vi "getResistance.vi"(5 "Uncertainty (%) Resistor":dbl=1.0, 6 "Uncertainty (%) Vin":dbl=1.0, 7 "Uncertainty (%) Vout":dbl=1.0, 8 "error in (no error)":errorcluster, 9 "V_in (V)":dbl=5.0, 10 "Resistor (ohms)":dbl=10000.0) -> (0 "error out":errorcluster, 2 "Uncertainty (%) Thermistor":dbl=3.0625, 3 "Resistance (ohms)":dbl=10000.0)   [LabVIEW 2013]
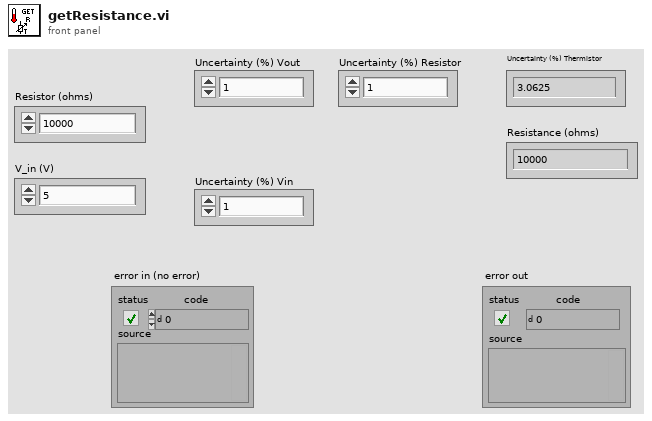
[diagram p1: front panel]
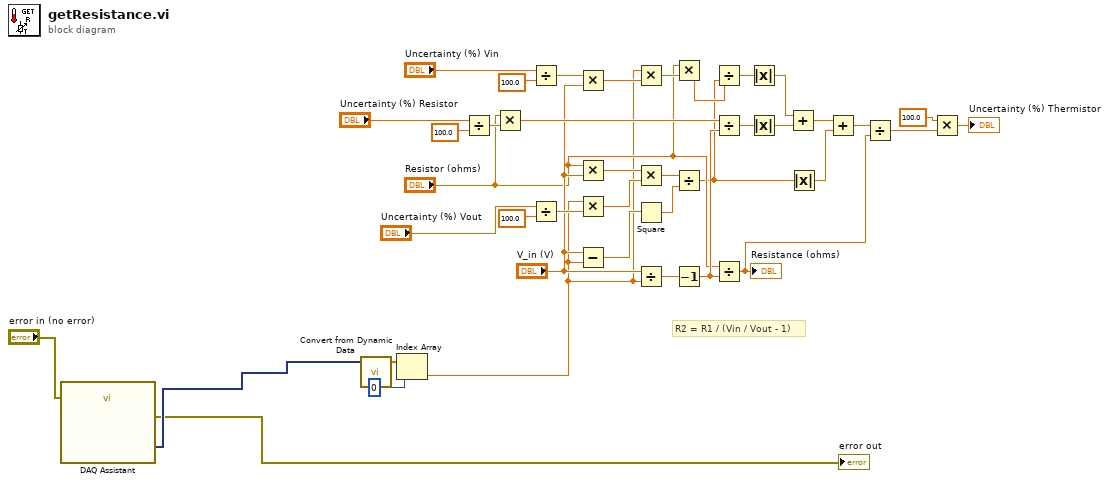
[diagram p0: block diagram]
diagram:
  # "R2 = R1 / (Vin / Vout - 1)"
  n1 = call "DAQ Assistant"("error in"="error in (no error)") -> ("data"=w2:dynamicdata, "error out"=→"error out":errorcluster)  [unwired: 16 in, 1 out]
  n2 = call "Convert from Dynamic Data"("Dynamic Data Type"=w2) -> ("Array"=w6:dbl[])  [unwired: 3 in]
  n3 = Index Array(array=w6, index=0) -> (element=w4:dbl)
  n4 = Divide(x="Uncertainty (%) Resistor", y=100.0) -> (x/y=w30:dbl)
  n5 = Multiply(x="Resistor (ohms)", y=w30) -> (x*y=w37:dbl)
  n6 = Divide(x="Uncertainty (%) Vin", y=100.0) -> (x/y=w22:dbl)
  n7 = Divide(x="Uncertainty (%) Vout", y=100.0) -> (x/y=w26:dbl)
  n8 = Multiply(x=w22, y="V_in (V)") -> (x*y=w21:dbl)
  n9 = Multiply(x="Resistor (ohms)", y="V_in (V)") -> (x*y=w35:dbl)
  n10 = Multiply(x=w4, y=w26) -> (x*y=w34:dbl)
  n11 = Subtract(x="V_in (V)", y=w4) -> (x-y=w36:dbl)
  n12 = Multiply(x=w4, y=w21) -> (x*y=w20:dbl)
  n13 = Multiply(x=w35, y=w34) -> (x*y=w33:dbl)
  n14 = Square(x=w36) -> (x^2=w32:dbl)
  n15 = Divide(x="V_in (V)", y=w4) -> (x/y=w40:dbl)
  n16 = Multiply(x="Resistor (ohms)", y=w20) -> (x*y=w18:dbl)
  n17 = Divide(x=w33, y=w32) -> (x/y=w17:dbl)
  n18 = Decrement(x=w40) -> (x-1=w39:dbl)
  n19 = Divide(x=w18, y=w17) -> (x/y=w16:dbl)
  n20 = Divide(x=w37, y=w39) -> (x/y=w38:dbl)
  n21 = Divide(x="Resistor (ohms)", y=w39) -> (x/y=w11:dbl)
  "Resistance (ohms)" <- w11
  n22 = Absolute Value(x=w16) -> (abs(x)=w15:dbl)
  n23 = Absolute Value(x=w38) -> (abs(x)=w14:dbl)
  n24 = Add(x=w15, y=w14) -> (x+y=w13:dbl)
  n25 = Absolute Value(x=w17) -> (abs(x)=w12:dbl)
  n26 = Add(x=w13, y=w12) -> (x+y=w10:dbl)
  n27 = Divide(x=w10, y=w11) -> (x/y=w8:dbl)
  n28 = Multiply(x=100.0, y=w8) -> (x*y=→"Uncertainty (%) Thermistor":dbl)
